vi "MNK_Z_Bridge_to_DSC.vi"(0 "description, string":refnum<k21>="ni.var.psp://housesoftheholy/MNK_18T/MNK_TC_Z_description", 1 "dbl var":refnum<k21>[](array[refnum])=["ni.var.psp://housesoftheholy/MNK_18T/MNK_Cstill_Z", "ni.var.psp://housesoftheholy/MNK_18T/MNK_CMN-187_Z", "ni.var.psp://housesoftheholy/MNK_18T/MNK_Cstill_T", "ni.var.psp://housesoftheholy/MNK_18T/MNK_CMN-187_T"], 2 "dbl":dbl[](array[numeric]), 5 "String In":string, 7 "calibration string":refnum<k21>="ni.var.psp://housesoftheholy/MNK_18T/MNK_TC_Z_calibration", 9 "String In 2":string) -> ()   [LabVIEW 2013]
panel:
  # "MNK Impedence Bridge to DSC"
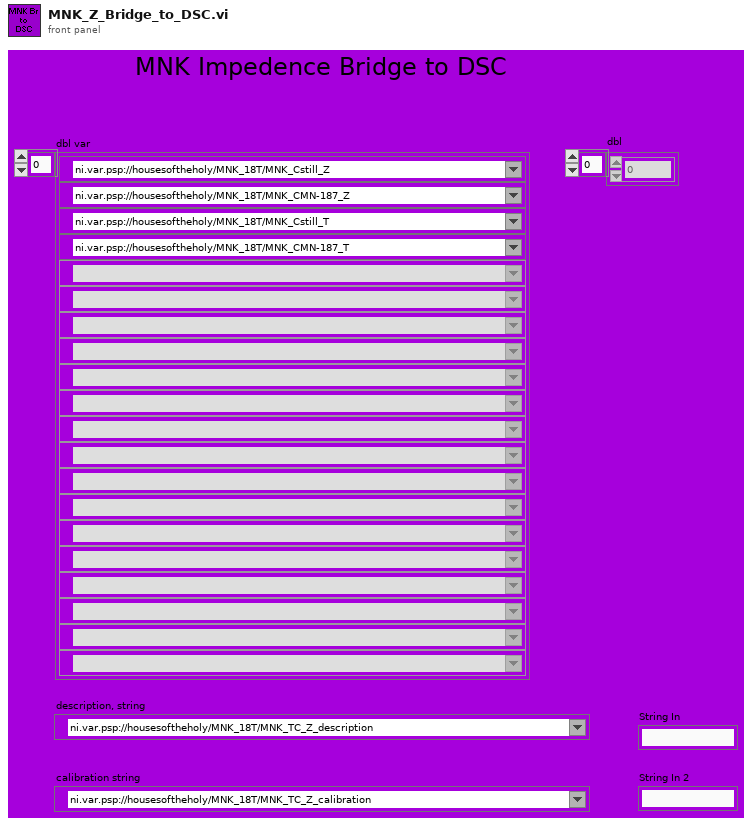
[diagram p1: front panel]
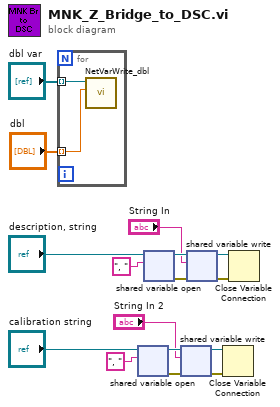
[diagram p0: block diagram]
diagram:
  n1 = for {
    tunnel: "dbl var" -> [w18] mode=indexing
    tunnel: "dbl" -> [w17] mode=indexing
    n2 = call "NetVarWrite_dbl.vi"("Numeric"=w17, "Refnum in"=w18) -> ()  [unwired: 10 in]
  }
  n3 = shared-variable-open("calibration string", ", " ("string")) -> (w13:refnum<k21>, w12:errorcluster)  [unwired: 2 in]
  n4 = shared-variable-open("description, string", ", " ("string")) -> (w8:refnum<k21>, w7:errorcluster)  [unwired: 2 in]
  n5 = shared-variable-write(w13, w12, "String In 2") -> (w14:refnum<k21>, w11:errorcluster)
  n6 = shared-variable-write(w8, w7, "String In") -> (w9:refnum<k21>, w6:errorcluster)
  n7 = Close Variable Connection(8:w11, 11:w14) -> ()  [unwired: 1 out]
  n8 = Close Variable Connection(8:w6, 11:w9) -> ()  [unwired: 1 out]
